vi "AUTO_Drive Straight.vi"(11 "Raw Yaw":dbl) -> (3 "X-Axis Motor Output":dbl)   [LabVIEW 2015]
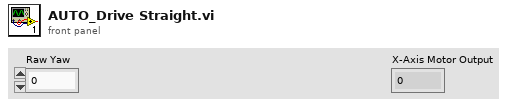
[diagram p1: front panel]
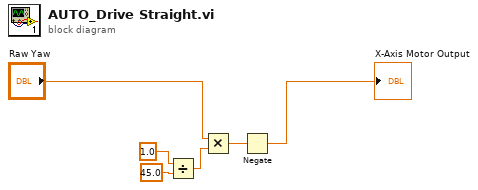
[diagram p0: block diagram]
diagram:
  n1 = Divide(x=1.0, y=45.0) -> (x/y=w6:dbl)
  n2 = Multiply(x="Raw Yaw", y=w6) -> (x*y=w3:dbl)
  n3 = Negate(x=w3) -> (-x=→"X-Axis Motor Output":dbl)
